vi "Read AppOutputData.vi"(8 "error in (no error)":errorcluster, 11 "RingdownPlugin in":refnum<class "RingdownPlugin.lvclass">) -> (0 "error out":errorcluster, 2 "AppOutputData":variant, 3 "RingdownPlugin out":refnum<class "RingdownPlugin.lvclass">)   [LabVIEW 2014, in "AppPlugins.lvlib" / "RingdownPlugin.lvclass"]
uses:
  RingdownPlugin.lvclass
  RingdownPlugin.lvclass/RingdownPlugin.ctl
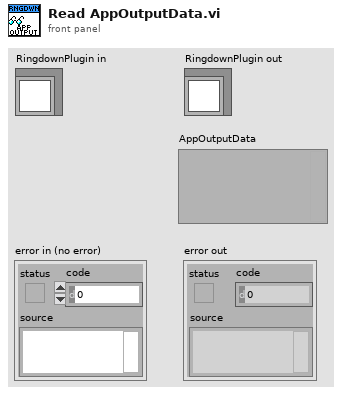
[diagram p1: front panel]
types:
  T1 = typedef "AppPlugins.lvlib/RingdownPlugin.lvclass/RingdownOutput.ctl" = cluster{"FramesPerSecond":dbl, "PronyEstimate":dbl[], "RingdownParameters":cluster{"Amplitude":dbl[], "Damping":dbl[], "Frequency":dbl[], "Phase":dbl[]}, "ReportingTime":dbl, "DataSize":u32, "InputSignal":dbl[]}
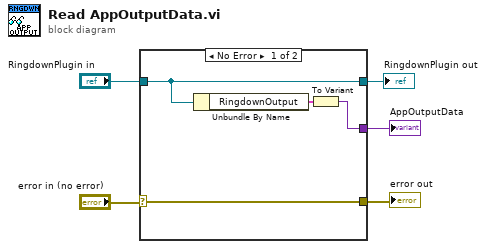
[diagram p0: block diagram]
diagram:
  n1 = case shown="No Error" "error in (no error)" {
    selector: "error in (no error)" -> [w6 w11]
    tunnel: [w7 _] -> w1
    tunnel: "RingdownPlugin in" -> [w8 w10]
    tunnel: [w6 w11] -> w3
    tunnel: [w8 w10] -> w2
    frame No Error {
      n2 = Unbundle By Name(w8) -> ("RingdownOutput"=w9:T1)
      n3 = To Variant(anything=w9) -> (Variant=w7:variant)
    }
    frame Error {
    }
  }
  "error out" <- w3
  "RingdownPlugin out" <- w2
  "AppOutputData" <- w1
